vi "Query Sequencer List Sample Rate.vi"(8 "error in (no error)":errorcluster, 9 "Index (0)":i32, 10 "Instance (1)":i32=1, 11 "VISA resource name":refnum<visa-resource-name>) -> (0 "error out":errorcluster, 2 "Sample Rate":dbl, 3 "VISA resource name out":refnum<visa-resource-name>)   [LabVIEW 2020, in "Rohde&Schwarz CMXP GPRF.lvlib"]
doc: "Queries the sample rate for the sequencer list entry with the selected Index.\n\nAttribute:\n-\n\nRemote-control command:\nSOURce:GPRF:GEN<i>:SEQuencer:LIST:SRATe?"
uses:
  <instrlib>/Rohde&Schwarz CMXP GPRF/Rohde&Schwarz CMXP GPRF.lvlib
  <instrlib>/Rohde&Schwarz CMXP GPRF/Private/rsidr_core.llb/rsidr_core.lvlib
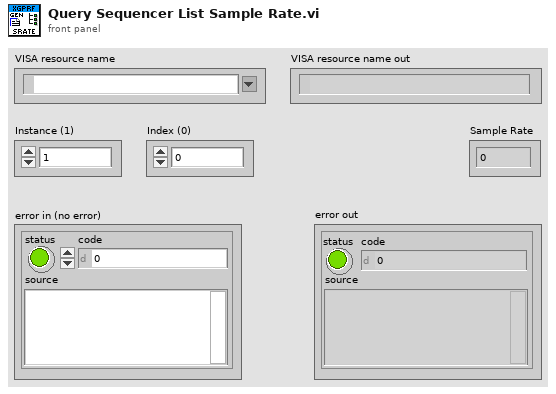
[diagram p1: front panel]
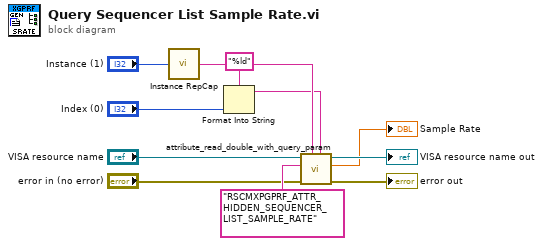
[diagram p0: block diagram]
diagram:
  n1 = call <instrlib>:"Instance RepCap.vi"("Instance in"="Instance (1)") -> ("Instance out"=w11:string)
  n2 = Format Into String(format string="%ld", "Index (0)") -> (resulting string=w8:string)  [unwired: 2 in, 1 out]
  n3 = call <instrlib>:"attribute_read_double_with_query_param.vi"("Query Parameter (None)"=w8, "Repeated Capability (\"\")"=w11, "error in"="error in (no error)", "Attribute ID"="RSCMXPGPRF_ATTR_HIDDEN_SEQUENCER_LIST_SAMPLE_RATE", "VISA resource name"="VISA resource name") -> ("error out"=→"error out":errorcluster, "Double out"=→"Sample Rate":dbl, "VISA resource name out"=→"VISA resource name out":refnum<visa-resource-name>)  [unwired: 4 in]
